vi "1L06-tb1D-bool-compare.vi"(10 "t2":bool[](array[boolean])=[TRUE, FALSE, FALSE, TRUE], 11 "t1":bool[](array[boolean])=[TRUE, FALSE, FALSE, TRUE]) -> (3 "t1 <>t2 ?":bool)   [LabVIEW 2010, in "lv_01.lvlib"]
doc: "t1 et t2 sont 2 tableaux de booléens. La sortie retourne VRAI (TRUE) si un seul des éléments des 2 tableaux est différent."
uses:
  lv_01.lvlib
panel:
  out "nombre":u32
  out "x != y ?":bool[](array[boolean])
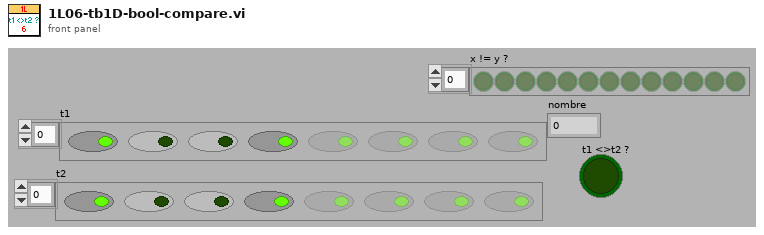
[diagram p1: front panel]
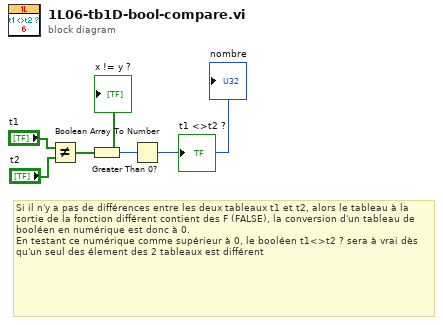
[diagram p0: block diagram]
diagram:
  # "Si il n'y a pas de différences entre les deux tableaux t1 et t2, alors le tableau à la sortie de la fonction différent contient des F (FALSE), la conversion d'un tableau de booléen en numérique est donc à 0.\nEn testant ce numérique comme supérieur à 0, le booléen t1<>t2 ? sera à vrai dès qu'un seul des élement des 2 tableaux est différent"
  n1 = Not Equal?(x="t1", y="t2") -> (x != y?=w3:bool[])
  "x != y ?" <- w3
  n2 = Boolean Array To Number(Boolean array=w3) -> (number=w2:u32)
  "nombre" <- w2
  n3 = Greater Than 0?(x=w2) -> (x > 0?=→"t1 <>t2 ?":bool)
